vi "fpga_ARC FIFO control.vi"(8 "Read FIFO":bool, 9 "write FIFO":bool, 10 "resample position":fxp<+,64,16> format="%.53g", 11 "frequency":fxp<+,32,8> format="%.27g") -> (0 "FIFO time out?":bool, 2 "resample position":fxp<+,64,16> format="%.53g", 3 "frequency":fxp<+,32,8> format="%.27g")   [LabVIEW 2011, in "NI_EP_Resample_FPGA.lvlib"]
uses:
  <vilib>/rvi/DataTransferAndStorage/Container/Common/niFpgaContainerState.ctl
  <vilib>/rvi/DataTransferAndStorage/Container/Common/niFpgaDataTypeControl.ctl
  <vilib>/rvi/DataTransferAndStorage/Container/Common/niFpgaContainerImplementationControl.ctl
  <vilib>/rvi/DataTransferAndStorage/Container/Common/niFpgaContainerArbitrationOptionsControl.ctl
  <vilib>/rvi/DataTransferAndStorage/Container/Common/niFpgaTransferTypeControl.ctl
  <vilib>/rvi/DataTransferAndStorage/Container/Common/niFpgaContainerInitializationParameters.ctl
  <vilib>/rvi/Memory/Memory_Types/niFpgaMemoryInterfaceConfiguration.ctl
  <vilib>/rvi/FIFO/Fifo_Types/niFpgaFifoControlLogicControl.ctl
  <vilib>/rvi/DataTransferAndStorage/Container/Common/niFpgaContainerMetaDataKey.ctl
  <vilib>/rvi/DataTransferAndStorage/Container/Common/niFpgaContainerGetUniqueNameForEmu.vi
  <vilib>/rvi/DataTransferAndStorage/Container/Common/niFpgaContainerSetEmuInfo.vi
  <vilib>/rvi/eio/common/nirviEmuReportErrorAndStop.vi
  <vilib>/rvi/FIFO/Fifo_Resource/nirvififoEmulationSetSize.vi
  <vilib>/rvi/LocalResourceManager/LocalResourceManager.xnode
  <vilib>/rvi/DataTransferAndStorage/Container/XNode/niFpgaContainer.xnode
  <vilib>/rvi/FIFO/Fifo_Resource/nirvififoEmulationWrite.vi
  <vilib>/rvi/FIFO/Fifo_Resource/nirvififoEmulationRead.vi
  <vilib>/addons/Electrical Power/PQ/Resampling/NI_EP_Resample_FPGA.lvlib
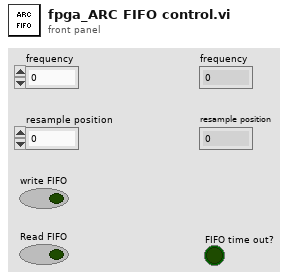
[diagram p1: front panel]
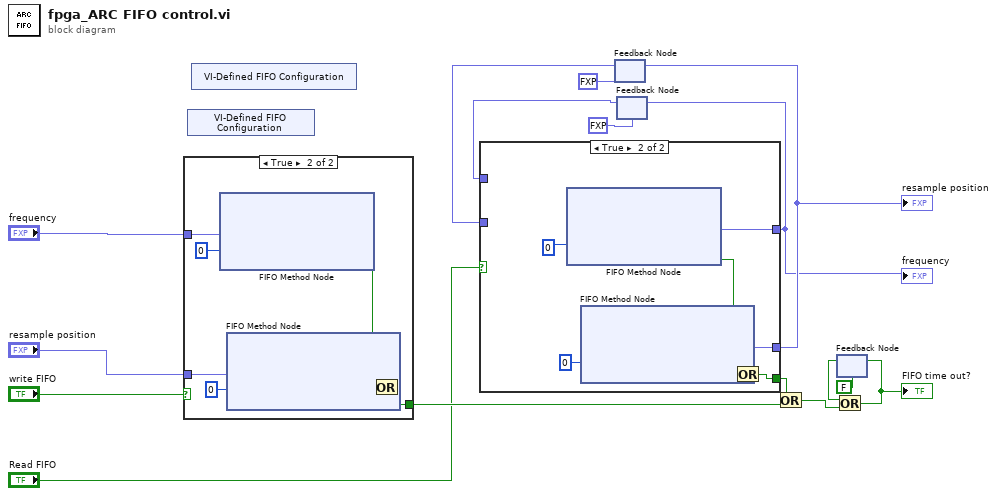
[diagram p0: block diagram]
diagram:
  n1 = case shown="True" "write FIFO" {
    tunnel: [_ w18] -> w16
    tunnel: "resample position" -> [_ w22]
    tunnel: "frequency" -> [_ w17]
    frame False {
    }
    frame True {
      n2 = xnode ("FIFO Method Node")("Element"=w17, "Timeout"=0) -> ("Timed Out?"=w19:bool)  [unwired: 1 in, 1 out]
      n3 = xnode ("FIFO Method Node")("Element"=w22, "Timeout"=0) -> ("Timed Out?"=w20:bool)  [unwired: 1 in, 1 out]
      n4 = Or(x=w19, y=w20) -> (x .or. y?=w18:bool)
    }
  }
  n5 = xnode "VI-Defined FIFO Configuration"() -> ()  [unwired: 1 out]
  n6 = xnode "VI-Defined FIFO Configuration"() -> ()  [unwired: 1 out]
  n7 = feedback #1(fxp<+,64,16> 0.0 ("Element")) -> (w14:fxp<+,64,16>)
  n8 = feedback #2(fxp<+,32,8> 0.0 ("Element")) -> (w12:fxp<+,32,8>)
  n9 = case shown="True" "Read FIFO" {
    tunnel: [w25 w31] -> w7
    tunnel: [_ w27] -> w15
    tunnel: w14 -> [w25 _]
    tunnel: [w24 w26] -> w5
    tunnel: w12 -> [w24 _]
    frame False {
    }
    frame True {
      n10 = xnode ("FIFO Method Node")("Timeout"=0) -> ("Element"=w26:fxp<+,32,8>, "Timed Out?"=w29:bool)  [unwired: 1 in, 1 out]
      n11 = xnode ("FIFO Method Node")("Timeout"=0) -> ("Element"=w31:fxp<+,64,16>, "Timed Out?"=w28:bool)  [unwired: 1 in, 1 out]
      n12 = Or(x=w29, y=w28) -> (x .or. y?=w27:bool)
    }
  }
  "frequency" <- w5
  "resample position" <- w7
  n13 = feedback-in #1(w7) -> ()
  n14 = feedback-in #2(w5) -> ()
  n15 = Or(x=w15, y=w16) -> (x .or. y?=w11:bool)
  n16 = feedback #3(FALSE) -> (w10:bool)
  n17 = Or(x=w10, y=w11) -> (x .or. y?=w8:bool)
  "FIFO time out?" <- w8
  n18 = feedback-in #3(w8) -> ()
